vi "COMWriteLine.vi"(8 "error in (no error)":errorcluster, 9 "String":string, 10 "Port ID":i32(ring)=2 items=["COM2"=2, "COM3"=3], 11 "SM1000-control in":T1) -> (0 "error out":errorcluster, 1 "Return string":string, 3 "SM1000-control out":T1)   [LabVIEW 2013, in "HardwareCharacterization.lvlib" / "HC-SM1000.lvclass"]
doc: "Writes the string argument to the COM port on the EC1000.\n\nThis operation is intended to permit out-of-band communication to serial port based automation devices or laser systems. The specified port-ID must have been opened with the command 'OpenCOMPort'.\n\nCommand: <\"COMWriteLine\">,<port-ID>,<string>,<timeout (ms)> or 18,<port-ID>,<string>,<timeout (ms)>\nReturns: \"ERROR_PORT_TIMEOUT\" on timeout"
uses:
  HC-SM1000.lvclass
  Object-reference.ctl
  HC-SM1000.lvclass/HC-SM1000.ctl
  Custom-errors.ctl
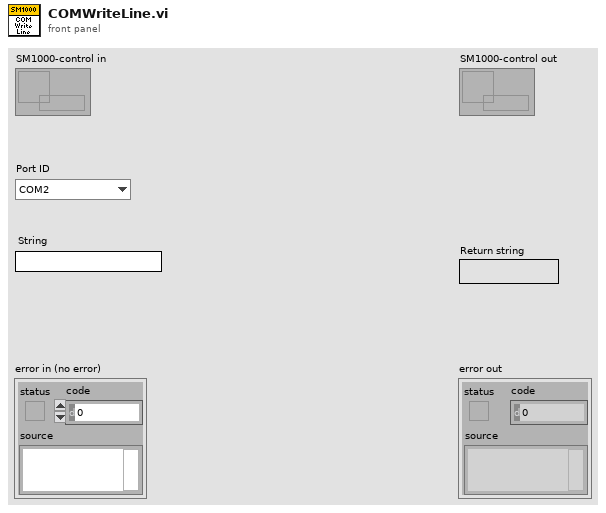
[diagram p1: front panel]
types:
  T1 = typedef "HardwareCharacterization.lvlib/HC-SM1000.lvclass/Object-reference.ctl" = refnum<data-value>
  T2 = typedef "HardwareCharacterization.lvlib/HC-SM1000.lvclass/Custom-errors.ctl" = enum16{"No error", "Not implemented", "Command not recognized", "Invalid input", "No connection", "Timeout", "Resource not loaded"}
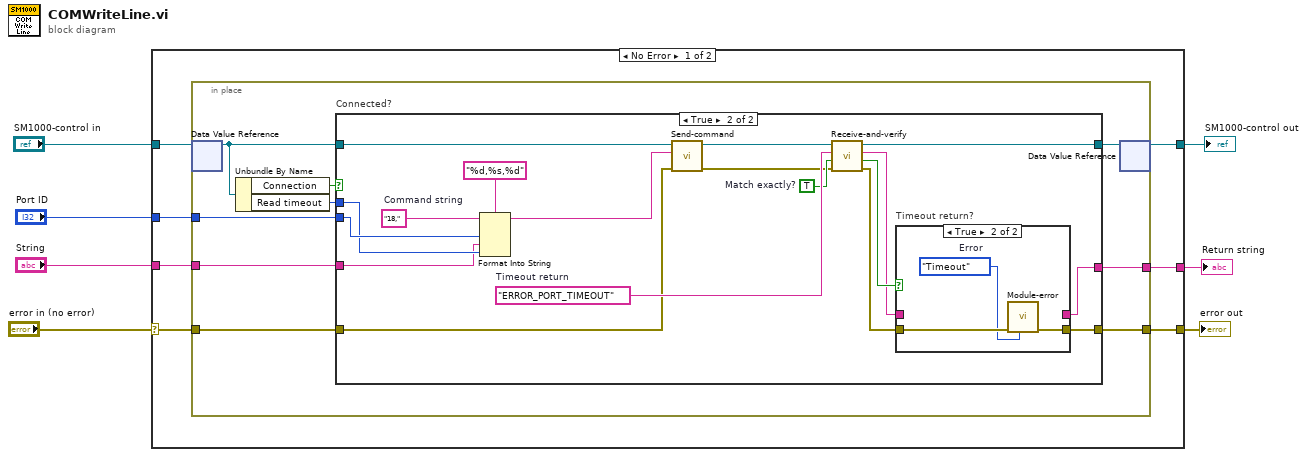
[diagram p0: block diagram]
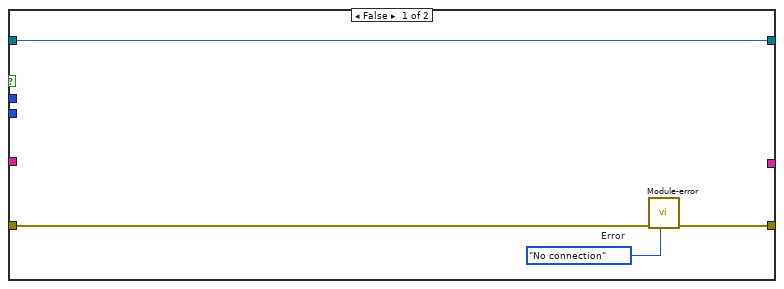
[diagram p2: hidden frame]
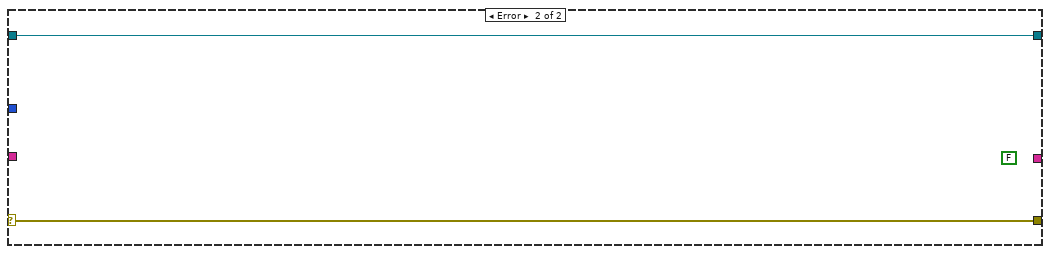
[diagram p4: hidden frame]
diagram:
  n1 = case shown="No Error" "error in (no error)" {
    selector: "error in (no error)" -> [w12 w52]
    tunnel: [w11 w52] -> w6
    tunnel: [w13 w51] -> w4
    tunnel: "SM1000-control in" -> [w14 w51]
    tunnel: "Port ID" -> [w10 _]
    tunnel: "String" -> [w9 _]
    tunnel: [w8 _] -> w1
    frame No Error {
      n2 = in-place {
        in-place-border: w12 -> [w23]
        in-place-border: [w20] -> w11
        in-place-border: w10 -> [w18]
        in-place-border: w9 -> [w16]
        in-place-border: [w15] -> w8
        n3 = in-place-dvr #1(w14) -> (w21:refnum<class "HC-SM1000.lvclass">)  [unwired: 1 out]
        n4 = Unbundle By Name(w21) -> ("Connection"=w22:bool, "Read timeout"=w17:i32)
        n5 = case "Connected?" shown="True" w22 {
          tunnel: w23 -> [w27 w38]
          tunnel: w21 -> [w25 w45]
          tunnel: [w26 w36] -> w20
          tunnel: [w25 w35] -> w19
          tunnel: w18 -> [_ w32]
          tunnel: w17 -> [_ w31]
          tunnel: w16 -> [_ w29]
          tunnel: [_ w28] -> w15
          frame False {
            w24 = Custom-errors."No connection"  # Error
            n6 = call "Module-error.vi"("Error"=w24, "error in (no error)"=w27) -> ("error out"=w26:errorcluster)  [unwired: 9 in]
          }
          frame True {
            w42 = TRUE  # Match exactly?
            w43 = "ERROR_PORT_TIMEOUT"  # Timeout return
            w34 = "18,"  # Command string
            n7 = Format Into String(format string="%d,%s,%d", initial string=w34, w32, w29, w31) -> (resulting string=w33:string)  [unwired: 1 in, 1 out]
            n8 = call "Send-command.vi"("error in (no error)"=w38, "Command string"=w33, "SM1000-control in"=w45) -> ("error out"=w41:errorcluster, "SM1000-control out"=w44:refnum<class "HC-SM1000.lvclass">)  [unwired: 7 in]
            n9 = call "Receive-and-verify.vi"("error in (no error)"=w41, "Match exactly?"=w42, "Expected return string"=w43, "SM1000-control in"=w44) -> ("error out"=w37:errorcluster, "Verified?"=w40:bool, "Return string"=w39:string, "SM1000-control out"=w35:refnum<class "HC-SM1000.lvclass">)  [unwired: 4 in]
            n10 = case "Timeout return?" shown="True" w40 {
              tunnel: w39 -> [w46 _]
              tunnel: w37 -> [w47 w49]
              tunnel: [w47 w50] -> w36
              tunnel: [w46 _] -> w28
              frame False {
              }
              frame True {
                w48 = Custom-errors."Timeout"  # Error
                n11 = call "Module-error.vi"("Error"=w48, "error in (no error)"=w49) -> ("error out"=w50:errorcluster)  [unwired: 9 in]
              }
            }
          }
        }
        n12 = in-place-dvr #1(w19) -> (w13:T1)  [unwired: 1 out]
      }
    }
    frame Error {
      (unwired) FALSE
    }
  }
  "error out" <- w6
  "SM1000-control out" <- w4
  "Return string" <- w1
